vi "initialiseDevice.vi"(8 "error in (no error)":errorcluster, 10 "deviceName":string, 11 "AtomChipHWC in":refnum<class "AtomChipHWC.lvclass">) -> (0 "error out":errorcluster, 3 "AtomChipHWC out":refnum<class "AtomChipHWC.lvclass">)   [LabVIEW 2011, in "Hardware.lvlib" / "HWControllers.lvlib" / "AtomChipHWC.lvclass"]
doc: "Initialise a hardware device. \nI.e. set its initial channel states etc."
uses:
  AtomChipHWC.lvclass
  AtomChipHWC.lvclass/AtomChipHWC.ctl
  Channels/VoltOutput/AnalogOutput.lvclass
  Channels/Digital/DigitalOutput.lvclass
  Channels/DDSOutput/Generic/DDSOutput.lvclass
  Network Controllers/NetworkCamera/NetworkCamera.lvclass
  HWController.lvclass
  Tools/DatabaseHelpers/DbConnection/DeviceDataBase/deviceDataBase.lvclass
  Network Controllers/CameraNetworkController/CameraNetworkController.lvclass
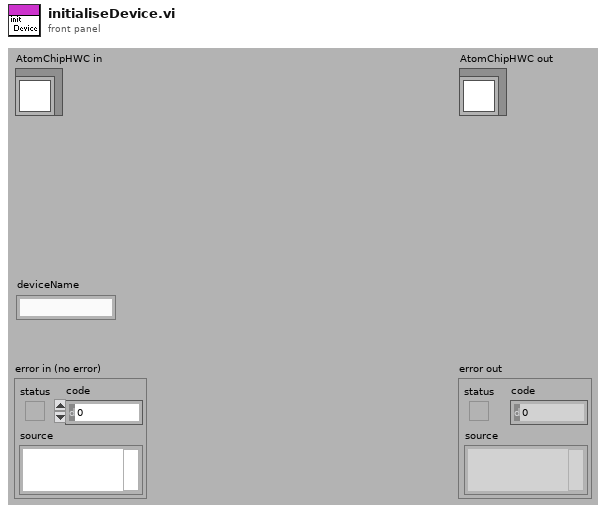
[diagram p1: front panel]
types:
  T1 = cluster{"VoltageLimit":dbl, "CurrentLimit":dbl}[]
  T2 = cluster{"Frequency(MHz)":dbl, "Amplitude":dbl, "Phase":dbl, "OutputForm":enum16{"Sine", "Square", "Triangle", "Arbitrary"}}[]
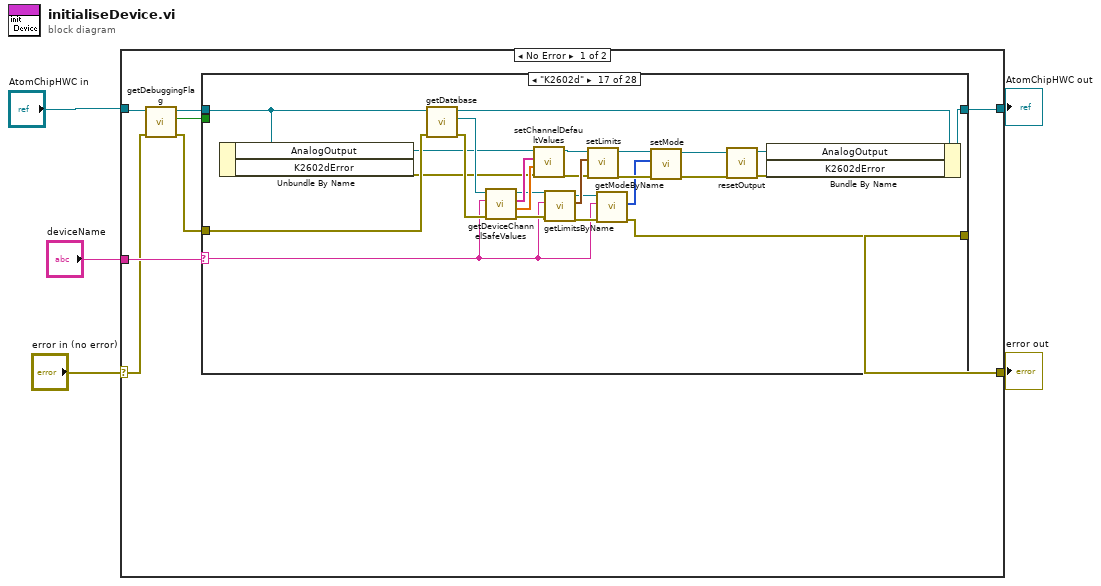
[diagram p0: block diagram]
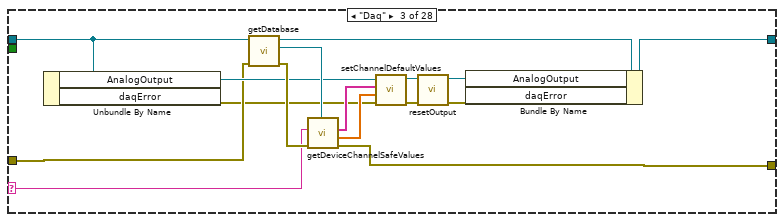
[diagram p4: hidden frame]
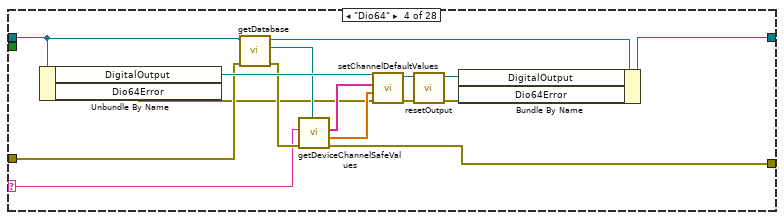
[diagram p5: hidden frame]
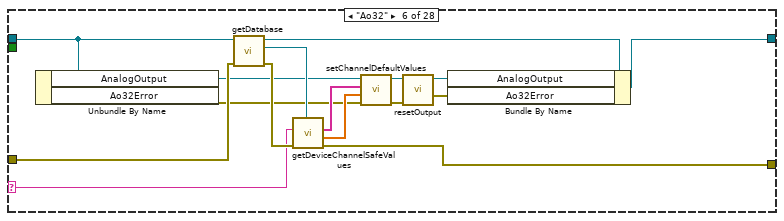
[diagram p7: hidden frame]
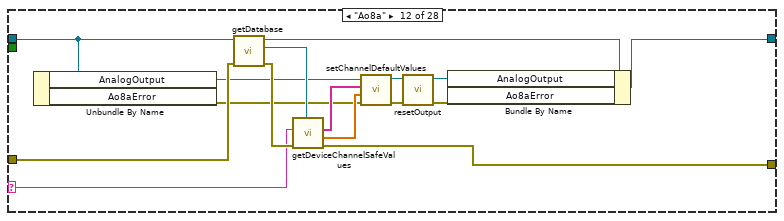
[diagram p13: hidden frame]
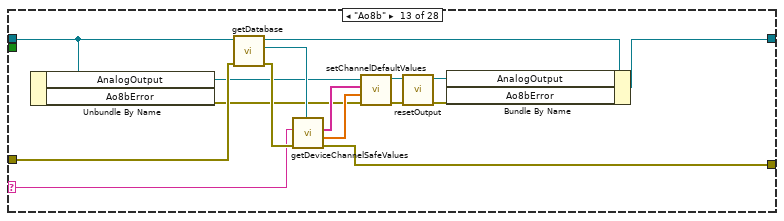
[diagram p14: hidden frame]
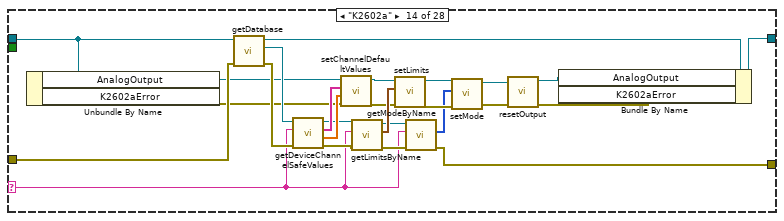
[diagram p15: hidden frame]
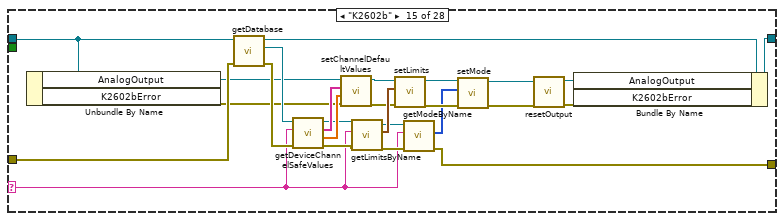
[diagram p16: hidden frame]
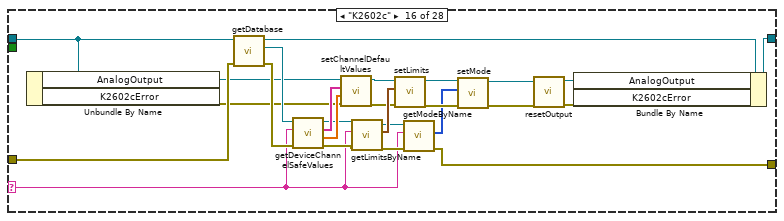
[diagram p17: hidden frame]
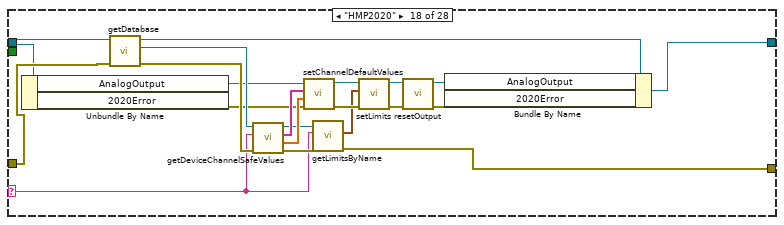
[diagram p18: hidden frame]
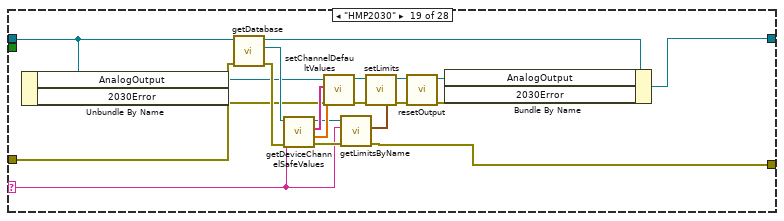
[diagram p19: hidden frame]
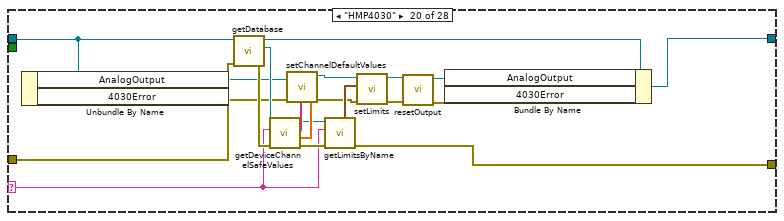
[diagram p20: hidden frame]
diagram:
  n1 = case shown="No Error" "error in (no error)" {
    selector: "error in (no error)" -> [w8 w374]
    tunnel: [w11 w374] -> w4
    tunnel: [w13 w373] -> w2
    tunnel: "AtomChipHWC in" -> [w10 w373]
    tunnel: "deviceName" -> [w12 _]
    frame No Error {
      n2 = call "getDebuggingFlag.vi"("error in (no error)"=w8, "HWController.lvclass in"=w10) -> ("error out"=w7:errorcluster, "debuggingFlag"=w6:bool, "HWController.lvclass out"=w9:refnum<class "AtomChipHWC.lvclass">)  [unwired: 7 in]
      n3 = case shown="\"K2602d\"" w12 {
        selector: w12 -> [_ _ w21 w40 _ w65 _ _ _ _ _ w91 w107 w112 w138 w164 w190 w220 w236 w257 w285 w302 w321 w339 _ _ _ _]
        tunnel: w9 -> [w15 w17 w24 w44 w50 w59 w69 w71 w73 w75 w77 w86 w101 w130 w156 w182 w208 w223 w251 w272 w291 w307 w325 w343 w350 w358 w365 w372]
        tunnel: [w15 w17 w22 w45 w50 w55 w69 w71 w73 w75 w77 w82 w97 w126 w152 w178 w204 w228 w247 w268 w289 w305 w323 w341 w348 w357 w364 w371] -> w13
        tunnel: w7 -> [w14 w16 w23 w37 w51 w64 w68 w70 w72 w74 w76 w90 w106 w133 w159 w185 w211 w232 w253 w274 w292 w308 w326 w344 w345 w356 w363 w370]
        tunnel: [w14 w16 w18 w34 w51 w52 w68 w70 w72 w74 w76 w79 w96 w110 w137 w163 w189 w219 w235 w256 w279 w295 w314 w332 w345 w356 w363 w370] -> w11
        tunnel: w6 -> [_ _ _ _ _ _ _ _ _ _ _ _ _ _ _ _ _ _ _ _ _ _ _ _ _ _ _ _]
        frame "No Hardware", Default {
        }
        frame "UsbDAQ" {
        }
        frame "Daq" {
          n4 = Unbundle By Name(w24) -> ("AnalogOutput"=w27:refnum<class "AnalogOutput.lvclass">, "daqError"=w20:errorcluster)
          n5 = call "getDatabase.vi"("error in (no error)"=w23, "HWController in"=w24) -> ("error out"=w32:errorcluster, "deviceDataBase"=w33:refnum<class "deviceDataBase.lvclass">, "HWController out"=w25:refnum<class "AtomChipHWC.lvclass">)  [unwired: 7 in]
          n6 = call "getDeviceChannelSafeValues.vi"("error in (no error)"=w32, "device_name"=w21, "deviceDataBase in"=w33) -> ("error out"=w18:errorcluster, "SafeVaues"=w31:dbl[], "ChannelAddresses"=w30:string[])  [unwired: 5 in, 1 out]
          n7 = call "setChannelDefaultValues.vi"("error in (no error)"=w20, "calibratedValues"=w31, "channel_addresses"=w30, "AnalogOutput in"=w27) -> ("error out"=w28:errorcluster, "AnalogOutput out"=w29:refnum<class "AnalogOutput.lvclass">)  [unwired: 6 in]
          n8 = call-dynamic "resetOutput.vi"("error in (no error)"=w28, "AnalogOutput in"=w29) -> ("error out"=w19:errorcluster, "AnalogOutput out"=w26:refnum<class "AnalogOutput.lvclass">)  [unwired: 8 in]
          n9 = Bundle By Name(cluster=w25, "AnalogOutput"=w26, "daqError"=w19) -> (w22:refnum<class "AtomChipHWC.lvclass">)
        }
        frame "Dio64" {
          n10 = Unbundle By Name(w44) -> ("DigitalOutput"=w49:refnum<class "DigitalOutput.lvclass">, "Dio64Error"=w36:errorcluster)
          n11 = call "getDatabase.vi"("error in (no error)"=w37, "HWController in"=w44) -> ("error out"=w41:errorcluster, "deviceDataBase"=w42:refnum<class "deviceDataBase.lvclass">, "HWController out"=w43:refnum<class "AtomChipHWC.lvclass">)  [unwired: 7 in]
          n12 = call "getDeviceChannelSafeValues.vi"("error in (no error)"=w41, "device_name"=w40, "deviceDataBase in"=w42) -> ("error out"=w34:errorcluster, "SafeVaues"=w38:dbl[], "ChannelAddresses"=w39:string[])  [unwired: 5 in, 1 out]
          n13 = call-dynamic "setChannelDefaultValues.vi"("error in (no error)"=w36, "calibratedValues"=w38, "channel_addresses"=w39, "DigitalOutput in"=w49) -> ("error out"=w47:errorcluster, "DigitalOutput out"=w48:refnum<class "DigitalOutput.lvclass">)  [unwired: 6 in]
          n14 = call-dynamic "resetOutput.vi"("error in (no error)"=w47, "DigitalOutput in"=w48) -> ("error out"=w35:errorcluster, "DigitalOutput out"=w46:refnum<class "DigitalOutput.lvclass">)  [unwired: 8 in]
          n15 = Bundle By Name(cluster=w43, "DigitalOutput"=w46, "Dio64Error"=w35) -> (w45:refnum<class "AtomChipHWC.lvclass">)
        }
        frame "Ao8" {
        }
        frame "Ao32" {
          n16 = Unbundle By Name(w59) -> ("AnalogOutput"=w58:refnum<class "AnalogOutput.lvclass">, "Ao32Error"=w54:errorcluster)
          n17 = call "getDatabase.vi"("error in (no error)"=w64, "HWController in"=w59) -> ("error out"=w66:errorcluster, "deviceDataBase"=w67:refnum<class "deviceDataBase.lvclass">, "HWController out"=w56:refnum<class "AtomChipHWC.lvclass">)  [unwired: 7 in]
          n18 = call "getDeviceChannelSafeValues.vi"("error in (no error)"=w66, "device_name"=w65, "deviceDataBase in"=w67) -> ("error out"=w52:errorcluster, "SafeVaues"=w63:dbl[], "ChannelAddresses"=w62:string[])  [unwired: 5 in, 1 out]
          n19 = call "setChannelDefaultValues.vi"("error in (no error)"=w54, "calibratedValues"=w63, "channel_addresses"=w62, "AnalogOutput in"=w58) -> ("error out"=w60:errorcluster, "AnalogOutput out"=w61:refnum<class "AnalogOutput.lvclass">)  [unwired: 6 in]
          n20 = call-dynamic "resetOutput.vi"("error in (no error)"=w60, "AnalogOutput in"=w61) -> ("error out"=w53:errorcluster, "AnalogOutput out"=w57:refnum<class "AnalogOutput.lvclass">)  [unwired: 8 in]
          n21 = Bundle By Name(cluster=w56, "AnalogOutput"=w57, "Ao32Error"=w53) -> (w55:refnum<class "AtomChipHWC.lvclass">)
        }
        frame "ArbWave" {
        }
        frame "ICCamera" {
        }
        frame "AndorIKon" {
        }
        frame "S1010" {
        }
        frame "C100" {
        }
        frame "Ao8a" {
          n22 = Unbundle By Name(w86) -> ("AnalogOutput"=w85:refnum<class "AnalogOutput.lvclass">, "Ao8aError"=w80:errorcluster)
          n23 = call "getDatabase.vi"("error in (no error)"=w90, "HWController in"=w86) -> ("error out"=w92:errorcluster, "deviceDataBase"=w93:refnum<class "deviceDataBase.lvclass">, "HWController out"=w83:refnum<class "AtomChipHWC.lvclass">)  [unwired: 7 in]
          n24 = call "getDeviceChannelSafeValues.vi"("error in (no error)"=w92, "device_name"=w91, "deviceDataBase in"=w93) -> ("error out"=w79:errorcluster, "SafeVaues"=w81:dbl[], "ChannelAddresses"=w89:string[])  [unwired: 5 in, 1 out]
          n25 = call "setChannelDefaultValues.vi"("error in (no error)"=w80, "calibratedValues"=w81, "channel_addresses"=w89, "AnalogOutput in"=w85) -> ("error out"=w87:errorcluster, "AnalogOutput out"=w88:refnum<class "AnalogOutput.lvclass">)  [unwired: 6 in]
          n26 = call-dynamic "resetOutput.vi"("error in (no error)"=w87, "AnalogOutput in"=w88) -> ("error out"=w78:errorcluster, "AnalogOutput out"=w84:refnum<class "AnalogOutput.lvclass">)  [unwired: 8 in]
          n27 = Bundle By Name(cluster=w83, "AnalogOutput"=w84, "Ao8aError"=w78) -> (w82:refnum<class "AtomChipHWC.lvclass">)
        }
        frame "Ao8b" {
          n28 = Unbundle By Name(w101) -> ("AnalogOutput"=w100:refnum<class "AnalogOutput.lvclass">, "Ao8bError"=w94:errorcluster)
          n29 = call "getDatabase.vi"("error in (no error)"=w106, "HWController in"=w101) -> ("error out"=w108:errorcluster, "deviceDataBase"=w109:refnum<class "deviceDataBase.lvclass">, "HWController out"=w98:refnum<class "AtomChipHWC.lvclass">)  [unwired: 7 in]
          n30 = call "getDeviceChannelSafeValues.vi"("error in (no error)"=w108, "device_name"=w107, "deviceDataBase in"=w109) -> ("error out"=w96:errorcluster, "SafeVaues"=w105:dbl[], "ChannelAddresses"=w104:string[])  [unwired: 5 in, 1 out]
          n31 = call "setChannelDefaultValues.vi"("error in (no error)"=w94, "calibratedValues"=w105, "channel_addresses"=w104, "AnalogOutput in"=w100) -> ("error out"=w102:errorcluster, "AnalogOutput out"=w103:refnum<class "AnalogOutput.lvclass">)  [unwired: 6 in]
          n32 = call-dynamic "resetOutput.vi"("error in (no error)"=w102, "AnalogOutput in"=w103) -> ("error out"=w95:errorcluster, "AnalogOutput out"=w99:refnum<class "AnalogOutput.lvclass">)  [unwired: 8 in]
          n33 = Bundle By Name(cluster=w98, "AnalogOutput"=w99, "Ao8bError"=w95) -> (w97:refnum<class "AtomChipHWC.lvclass">)
        }
        frame "K2602a" {
          n34 = Unbundle By Name(w130) -> ("AnalogOutput"=w129:refnum<class "AnalogOutput.lvclass">, "K2602aError"=w124:errorcluster)
          n35 = call "getDatabase.vi"("error in (no error)"=w133, "HWController in"=w130) -> ("error out"=w134:errorcluster, "deviceDataBase"=w135:refnum<class "deviceDataBase.lvclass">, "HWController out"=w127:refnum<class "AtomChipHWC.lvclass">)  [unwired: 7 in]
          n36 = call "getDeviceChannelSafeValues.vi"("error in (no error)"=w134, "device_name"=w112, "deviceDataBase in"=w135) -> ("error out"=w122:errorcluster, "SafeVaues"=w132:dbl[], "ChannelAddresses"=w131:string[], "deviceDataBase out"=w123:refnum<class "deviceDataBase.lvclass">)  [unwired: 5 in]
          n37 = call "setChannelDefaultValues.vi"("error in (no error)"=w124, "calibratedValues"=w132, "channel_addresses"=w131, "AnalogOutput in"=w129) -> ("error out"=w119:errorcluster, "AnalogOutput out"=w121:refnum<class "AnalogOutput.lvclass">)  [unwired: 6 in]
          n38 = call "getLimitsByName.vi"("error in (no error)"=w122, "device_name"=w112, "deviceDataBase in"=w123) -> ("error out"=w113:errorcluster, "Limits"=w120:T1, "deviceDataBase out"=w114:refnum<class "deviceDataBase.lvclass">)  [unwired: 6 in]
          n39 = call "setLimits.vi"("error in (no error)"=w119, "Limits"=w120, "AnalogOutput in"=w121) -> ("error out"=w115:errorcluster, "AnalogOutput out"=w118:refnum<class "AnalogOutput.lvclass">)  [unwired: 7 in]
          n40 = call "getModeByName.vi"("error in (no error)"=w113, "device_name"=w112, "deviceDataBase in"=w114) -> ("error out"=w110:errorcluster, "mode"=w111:enum16{"current", "voltage"}[])  [unwired: 6 in, 1 out]
          n41 = call "setMode.vi"("error in (no error)"=w115, "mode"=w111, "AnalogOutput in"=w118) -> ("error out"=w116:errorcluster, "AnalogOutput out"=w117:refnum<class "AnalogOutput.lvclass">)  [unwired: 7 in]
          n42 = call-dynamic "resetOutput.vi"("error in (no error)"=w116, "AnalogOutput in"=w117) -> ("error out"=w125:errorcluster, "AnalogOutput out"=w128:refnum<class "AnalogOutput.lvclass">)  [unwired: 8 in]
          n43 = Bundle By Name(cluster=w127, "AnalogOutput"=w128, "K2602aError"=w125) -> (w126:refnum<class "AtomChipHWC.lvclass">)
        }
        frame "K2602b" {
          n44 = Unbundle By Name(w156) -> ("AnalogOutput"=w155:refnum<class "AnalogOutput.lvclass">, "K2602bError"=w150:errorcluster)
          n45 = call "getDatabase.vi"("error in (no error)"=w159, "HWController in"=w156) -> ("error out"=w160:errorcluster, "deviceDataBase"=w161:refnum<class "deviceDataBase.lvclass">, "HWController out"=w153:refnum<class "AtomChipHWC.lvclass">)  [unwired: 7 in]
          n46 = call "getDeviceChannelSafeValues.vi"("error in (no error)"=w160, "device_name"=w138, "deviceDataBase in"=w161) -> ("error out"=w148:errorcluster, "SafeVaues"=w158:dbl[], "ChannelAddresses"=w157:string[], "deviceDataBase out"=w149:refnum<class "deviceDataBase.lvclass">)  [unwired: 5 in]
          n47 = call "setChannelDefaultValues.vi"("error in (no error)"=w150, "calibratedValues"=w158, "channel_addresses"=w157, "AnalogOutput in"=w155) -> ("error out"=w145:errorcluster, "AnalogOutput out"=w147:refnum<class "AnalogOutput.lvclass">)  [unwired: 6 in]
          n48 = call "getLimitsByName.vi"("error in (no error)"=w148, "device_name"=w138, "deviceDataBase in"=w149) -> ("error out"=w140:errorcluster, "Limits"=w146:T1, "deviceDataBase out"=w139:refnum<class "deviceDataBase.lvclass">)  [unwired: 6 in]
          n49 = call "setLimits.vi"("error in (no error)"=w145, "Limits"=w146, "AnalogOutput in"=w147) -> ("error out"=w143:errorcluster, "AnalogOutput out"=w144:refnum<class "AnalogOutput.lvclass">)  [unwired: 7 in]
          n50 = call "getModeByName.vi"("error in (no error)"=w140, "device_name"=w138, "deviceDataBase in"=w139) -> ("error out"=w137:errorcluster, "mode"=w136:enum16{"current", "voltage"}[])  [unwired: 6 in, 1 out]
          n51 = call "setMode.vi"("error in (no error)"=w143, "mode"=w136, "AnalogOutput in"=w144) -> ("error out"=w142:errorcluster, "AnalogOutput out"=w141:refnum<class "AnalogOutput.lvclass">)  [unwired: 7 in]
          n52 = call-dynamic "resetOutput.vi"("error in (no error)"=w142, "AnalogOutput in"=w141) -> ("error out"=w151:errorcluster, "AnalogOutput out"=w154:refnum<class "AnalogOutput.lvclass">)  [unwired: 8 in]
          n53 = Bundle By Name(cluster=w153, "AnalogOutput"=w154, "K2602bError"=w151) -> (w152:refnum<class "AtomChipHWC.lvclass">)
        }
        frame "K2602c" {
          n54 = Unbundle By Name(w182) -> ("AnalogOutput"=w181:refnum<class "AnalogOutput.lvclass">, "K2602cError"=w176:errorcluster)
          n55 = call "getDatabase.vi"("error in (no error)"=w185, "HWController in"=w182) -> ("error out"=w186:errorcluster, "deviceDataBase"=w187:refnum<class "deviceDataBase.lvclass">, "HWController out"=w179:refnum<class "AtomChipHWC.lvclass">)  [unwired: 7 in]
          n56 = call "getDeviceChannelSafeValues.vi"("error in (no error)"=w186, "device_name"=w164, "deviceDataBase in"=w187) -> ("error out"=w174:errorcluster, "SafeVaues"=w184:dbl[], "ChannelAddresses"=w183:string[], "deviceDataBase out"=w175:refnum<class "deviceDataBase.lvclass">)  [unwired: 5 in]
          n57 = call "setChannelDefaultValues.vi"("error in (no error)"=w176, "calibratedValues"=w184, "channel_addresses"=w183, "AnalogOutput in"=w181) -> ("error out"=w171:errorcluster, "AnalogOutput out"=w173:refnum<class "AnalogOutput.lvclass">)  [unwired: 6 in]
          n58 = call "getLimitsByName.vi"("error in (no error)"=w174, "device_name"=w164, "deviceDataBase in"=w175) -> ("error out"=w166:errorcluster, "Limits"=w172:T1, "deviceDataBase out"=w165:refnum<class "deviceDataBase.lvclass">)  [unwired: 6 in]
          n59 = call "setLimits.vi"("error in (no error)"=w171, "Limits"=w172, "AnalogOutput in"=w173) -> ("error out"=w169:errorcluster, "AnalogOutput out"=w170:refnum<class "AnalogOutput.lvclass">)  [unwired: 7 in]
          n60 = call "getModeByName.vi"("error in (no error)"=w166, "device_name"=w164, "deviceDataBase in"=w165) -> ("error out"=w163:errorcluster, "mode"=w162:enum16{"current", "voltage"}[])  [unwired: 6 in, 1 out]
          n61 = call "setMode.vi"("error in (no error)"=w169, "mode"=w162, "AnalogOutput in"=w170) -> ("error out"=w168:errorcluster, "AnalogOutput out"=w167:refnum<class "AnalogOutput.lvclass">)  [unwired: 7 in]
          n62 = call-dynamic "resetOutput.vi"("error in (no error)"=w168, "AnalogOutput in"=w167) -> ("error out"=w177:errorcluster, "AnalogOutput out"=w180:refnum<class "AnalogOutput.lvclass">)  [unwired: 8 in]
          n63 = Bundle By Name(cluster=w179, "AnalogOutput"=w180, "K2602cError"=w177) -> (w178:refnum<class "AtomChipHWC.lvclass">)
        }
        frame "K2602d" {
          n64 = Unbundle By Name(w208) -> ("AnalogOutput"=w207:refnum<class "AnalogOutput.lvclass">, "K2602dError"=w202:errorcluster)
          n65 = call "getDatabase.vi"("error in (no error)"=w211, "HWController in"=w208) -> ("error out"=w212:errorcluster, "deviceDataBase"=w213:refnum<class "deviceDataBase.lvclass">, "HWController out"=w205:refnum<class "AtomChipHWC.lvclass">)  [unwired: 7 in]
          n66 = call "getDeviceChannelSafeValues.vi"("error in (no error)"=w212, "device_name"=w190, "deviceDataBase in"=w213) -> ("error out"=w200:errorcluster, "SafeVaues"=w210:dbl[], "ChannelAddresses"=w209:string[], "deviceDataBase out"=w201:refnum<class "deviceDataBase.lvclass">)  [unwired: 5 in]
          n67 = call "setChannelDefaultValues.vi"("error in (no error)"=w202, "calibratedValues"=w210, "channel_addresses"=w209, "AnalogOutput in"=w207) -> ("error out"=w197:errorcluster, "AnalogOutput out"=w199:refnum<class "AnalogOutput.lvclass">)  [unwired: 6 in]
          n68 = call "getLimitsByName.vi"("error in (no error)"=w200, "device_name"=w190, "deviceDataBase in"=w201) -> ("error out"=w192:errorcluster, "Limits"=w198:T1, "deviceDataBase out"=w191:refnum<class "deviceDataBase.lvclass">)  [unwired: 6 in]
          n69 = call "setLimits.vi"("error in (no error)"=w197, "Limits"=w198, "AnalogOutput in"=w199) -> ("error out"=w195:errorcluster, "AnalogOutput out"=w196:refnum<class "AnalogOutput.lvclass">)  [unwired: 7 in]
          n70 = call "getModeByName.vi"("error in (no error)"=w192, "device_name"=w190, "deviceDataBase in"=w191) -> ("error out"=w189:errorcluster, "mode"=w188:enum16{"current", "voltage"}[])  [unwired: 6 in, 1 out]
          n71 = call "setMode.vi"("error in (no error)"=w195, "mode"=w188, "AnalogOutput in"=w196) -> ("error out"=w194:errorcluster, "AnalogOutput out"=w193:refnum<class "AnalogOutput.lvclass">)  [unwired: 7 in]
          n72 = call-dynamic "resetOutput.vi"("error in (no error)"=w194, "AnalogOutput in"=w193) -> ("error out"=w203:errorcluster, "AnalogOutput out"=w206:refnum<class "AnalogOutput.lvclass">)  [unwired: 8 in]
          n73 = Bundle By Name(cluster=w205, "AnalogOutput"=w206, "K2602dError"=w203) -> (w204:refnum<class "AtomChipHWC.lvclass">)
        }
        frame "HMP2020" {
          n74 = Unbundle By Name(w223) -> ("AnalogOutput"=w230:refnum<class "AnalogOutput.lvclass">, "2020Error"=w226:errorcluster)
          n75 = call "getDatabase.vi"("error in (no error)"=w232, "HWController in"=w223) -> ("error out"=w233:errorcluster, "deviceDataBase"=w234:refnum<class "deviceDataBase.lvclass">, "HWController out"=w224:refnum<class "AtomChipHWC.lvclass">)  [unwired: 7 in]
          n76 = call "getDeviceChannelSafeValues.vi"("error in (no error)"=w233, "device_name"=w220, "deviceDataBase in"=w234) -> ("error out"=w221:errorcluster, "SafeVaues"=w227:dbl[], "ChannelAddresses"=w231:string[], "deviceDataBase out"=w222:refnum<class "deviceDataBase.lvclass">)  [unwired: 5 in]
          n77 = call "setChannelDefaultValues.vi"("error in (no error)"=w226, "calibratedValues"=w227, "channel_addresses"=w231, "AnalogOutput in"=w230) -> ("error out"=w216:errorcluster, "AnalogOutput out"=w218:refnum<class "AnalogOutput.lvclass">)  [unwired: 6 in]
          n78 = call "getLimitsByName.vi"("error in (no error)"=w221, "device_name"=w220, "deviceDataBase in"=w222) -> ("error out"=w219:errorcluster, "Limits"=w214:T1)  [unwired: 6 in, 1 out]
          n79 = call "setLimits.vi"("error in (no error)"=w216, "Limits"=w214, "AnalogOutput in"=w218) -> ("error out"=w215:errorcluster, "AnalogOutput out"=w217:refnum<class "AnalogOutput.lvclass">)  [unwired: 7 in]
          n80 = call-dynamic "resetOutput.vi"("error in (no error)"=w215, "AnalogOutput in"=w217) -> ("error out"=w225:errorcluster, "AnalogOutput out"=w229:refnum<class "AnalogOutput.lvclass">)  [unwired: 8 in]
          n81 = Bundle By Name(cluster=w224, "AnalogOutput"=w229, "2020Error"=w225) -> (w228:refnum<class "AtomChipHWC.lvclass">)
        }
        frame "HMP2030" {
          n82 = Unbundle By Name(w251) -> ("AnalogOutput"=w250:refnum<class "AnalogOutput.lvclass">, "2030Error"=w245:errorcluster)
          n83 = call "getDatabase.vi"("error in (no error)"=w253, "HWController in"=w251) -> ("error out"=w254:errorcluster, "deviceDataBase"=w255:refnum<class "deviceDataBase.lvclass">, "HWController out"=w248:refnum<class "AtomChipHWC.lvclass">)  [unwired: 7 in]
          n84 = call "getDeviceChannelSafeValues.vi"("error in (no error)"=w254, "device_name"=w236, "deviceDataBase in"=w255) -> ("error out"=w237:errorcluster, "SafeVaues"=w246:dbl[], "ChannelAddresses"=w252:string[], "deviceDataBase out"=w238:refnum<class "deviceDataBase.lvclass">)  [unwired: 5 in]
          n85 = call "setChannelDefaultValues.vi"("error in (no error)"=w245, "calibratedValues"=w246, "channel_addresses"=w252, "AnalogOutput in"=w250) -> ("error out"=w239:errorcluster, "AnalogOutput out"=w242:refnum<class "AnalogOutput.lvclass">)  [unwired: 6 in]
          n86 = call "getLimitsByName.vi"("error in (no error)"=w237, "device_name"=w236, "deviceDataBase in"=w238) -> ("error out"=w235:errorcluster, "Limits"=w243:T1)  [unwired: 6 in, 1 out]
          n87 = call "setLimits.vi"("error in (no error)"=w239, "Limits"=w243, "AnalogOutput in"=w242) -> ("error out"=w240:errorcluster, "AnalogOutput out"=w241:refnum<class "AnalogOutput.lvclass">)  [unwired: 7 in]
          n88 = call-dynamic "resetOutput.vi"("error in (no error)"=w240, "AnalogOutput in"=w241) -> ("error out"=w244:errorcluster, "AnalogOutput out"=w249:refnum<class "AnalogOutput.lvclass">)  [unwired: 8 in]
          n89 = Bundle By Name(cluster=w248, "AnalogOutput"=w249, "2030Error"=w244) -> (w247:refnum<class "AtomChipHWC.lvclass">)
        }
        frame "HMP4030" {
          n90 = Unbundle By Name(w272) -> ("AnalogOutput"=w271:refnum<class "AnalogOutput.lvclass">, "4030Error"=w266:errorcluster)
          n91 = call "getDatabase.vi"("error in (no error)"=w274, "HWController in"=w272) -> ("error out"=w275:errorcluster, "deviceDataBase"=w276:refnum<class "deviceDataBase.lvclass">, "HWController out"=w269:refnum<class "AtomChipHWC.lvclass">)  [unwired: 7 in]
          n92 = call "getDeviceChannelSafeValues.vi"("error in (no error)"=w275, "device_name"=w257, "deviceDataBase in"=w276) -> ("error out"=w259:errorcluster, "SafeVaues"=w267:dbl[], "ChannelAddresses"=w273:string[], "deviceDataBase out"=w258:refnum<class "deviceDataBase.lvclass">)  [unwired: 5 in]
          n93 = call "setChannelDefaultValues.vi"("error in (no error)"=w266, "calibratedValues"=w267, "channel_addresses"=w273, "AnalogOutput in"=w271) -> ("error out"=w260:errorcluster, "AnalogOutput out"=w263:refnum<class "AnalogOutput.lvclass">)  [unwired: 6 in]
          n94 = call "getLimitsByName.vi"("error in (no error)"=w259, "device_name"=w257, "deviceDataBase in"=w258) -> ("error out"=w256:errorcluster, "Limits"=w264:T1)  [unwired: 6 in, 1 out]
          n95 = call "setLimits.vi"("error in (no error)"=w260, "Limits"=w264, "AnalogOutput in"=w263) -> ("error out"=w261:errorcluster, "AnalogOutput out"=w262:refnum<class "AnalogOutput.lvclass">)  [unwired: 7 in]
          n96 = call-dynamic "resetOutput.vi"("error in (no error)"=w261, "AnalogOutput in"=w262) -> ("error out"=w265:errorcluster, "AnalogOutput out"=w270:refnum<class "AnalogOutput.lvclass">)  [unwired: 8 in]
          n97 = Bundle By Name(cluster=w269, "AnalogOutput"=w270, "4030Error"=w265) -> (w268:refnum<class "AtomChipHWC.lvclass">)
        }
        frame "SpinCoreDDS0" {
          n98 = Unbundle By Name(w291) -> ("DDSOutput"=w288:refnum<class "DDSOutput.lvclass">, "DDS0Error"=w278:errorcluster)
          n99 = call "getDatabase.vi"("error in (no error)"=w292, "HWController in"=w291) -> ("error out"=w287:errorcluster, "deviceDataBase"=w286:refnum<class "deviceDataBase.lvclass">, "HWController out"=w290:refnum<class "AtomChipHWC.lvclass">)  [unwired: 7 in]
          n100 = call "getRfChannelSafeStates.vi"("error in (no error)"=w287, "deviceName"=w285, "deviceDataBase in"=w286) -> ("error out"=w279:errorcluster, "safestates"=w280:T2, "ChannelAddresses"=w281:string[])  [unwired: 5 in, 1 out]
          n101 = call-dynamic "setChannelDefaults.vi"("error in (no error)"=w278, "Data"=w280, "physicalChannels"=w281, "DDSOutput in"=w288) -> ("error out"=w282:errorcluster, "DDSOutput out"=w284:refnum<class "DDSOutput.lvclass">)  [unwired: 6 in]
          n102 = call-dynamic "resetOutput.vi"("error in (no error)"=w282, "DDSOutput in"=w284) -> ("error out"=w277:errorcluster, "DDSOutput out"=w283:refnum<class "DDSOutput.lvclass">)  [unwired: 8 in]
          n103 = Bundle By Name(cluster=w290, "DDSOutput"=w283, "DDS0Error"=w277) -> (w289:refnum<class "AtomChipHWC.lvclass">)
        }
        frame "SpinCoreDDS1" {
          n104 = Unbundle By Name(w307) -> ("DDSOutput"=w304:refnum<class "DDSOutput.lvclass">, "DDS1Error"=w294:errorcluster)
          n105 = call "getDatabase.vi"("error in (no error)"=w308, "HWController in"=w307) -> ("error out"=w303:errorcluster, "deviceDataBase"=w301:refnum<class "deviceDataBase.lvclass">, "HWController out"=w306:refnum<class "AtomChipHWC.lvclass">)  [unwired: 7 in]
          n106 = call "getRfChannelSafeStates.vi"("error in (no error)"=w303, "deviceName"=w302, "deviceDataBase in"=w301) -> ("error out"=w295:errorcluster, "safestates"=w299:T2, "ChannelAddresses"=w300:string[])  [unwired: 5 in, 1 out]
          n107 = call-dynamic "setChannelDefaults.vi"("error in (no error)"=w294, "Data"=w299, "physicalChannels"=w300, "DDSOutput in"=w304) -> ("error out"=w296:errorcluster, "DDSOutput out"=w298:refnum<class "DDSOutput.lvclass">)  [unwired: 6 in]
          n108 = call-dynamic "resetOutput.vi"("error in (no error)"=w296, "DDSOutput in"=w298) -> ("error out"=w293:errorcluster, "DDSOutput out"=w297:refnum<class "DDSOutput.lvclass">)  [unwired: 8 in]
          n109 = Bundle By Name(cluster=w306, "DDSOutput"=w297, "DDS1Error"=w293) -> (w305:refnum<class "AtomChipHWC.lvclass">)
        }
        frame "k3390" {
          n110 = Unbundle By Name(w325) -> ("DDSOutput"=w311:refnum<class "DDSOutput.lvclass">, "DDS1Error"=w309:errorcluster)
          n111 = call "getDatabase.vi"("error in (no error)"=w326, "HWController in"=w325) -> ("error out"=w322:errorcluster, "deviceDataBase"=w320:refnum<class "deviceDataBase.lvclass">, "HWController out"=w324:refnum<class "AtomChipHWC.lvclass">)  [unwired: 7 in]
          n112 = call "getRfChannelSafeStates.vi"("error in (no error)"=w322, "deviceName"=w321, "deviceDataBase in"=w320) -> ("error out"=w314:errorcluster, "safestates"=w318:T2, "ChannelAddresses"=w319:string[])  [unwired: 5 in, 1 out]
          n113 = call-dynamic "initialise.vi"("error in (no error)"=w309, "DDSOutput in"=w311) -> ("error out"=w310:errorcluster, "DDSOutput out"=w312:refnum<class "DDSOutput.lvclass">)  [unwired: 8 in]
          n114 = call-dynamic "setChannelDefaults.vi"("error in (no error)"=w310, "Data"=w318, "physicalChannels"=w319, "DDSOutput in"=w312) -> ("error out"=w315:errorcluster, "DDSOutput out"=w317:refnum<class "DDSOutput.lvclass">)  [unwired: 6 in]
          n115 = call-dynamic "resetOutput.vi"("error in (no error)"=w315, "DDSOutput in"=w317) -> ("error out"=w313:errorcluster, "DDSOutput out"=w316:refnum<class "DDSOutput.lvclass">)  [unwired: 8 in]
          n116 = Bundle By Name(cluster=w324, "DDSOutput"=w316, "DDS1Error"=w313) -> (w323:refnum<class "AtomChipHWC.lvclass">)
        }
        frame "CQTDDS0" {
          n117 = Unbundle By Name(w343) -> ("DDSOutput"=w329:refnum<class "DDSOutput.lvclass">, "DDS0Error"=w327:errorcluster)
          n118 = call "getDatabase.vi"("error in (no error)"=w344, "HWController in"=w343) -> ("error out"=w340:errorcluster, "deviceDataBase"=w338:refnum<class "deviceDataBase.lvclass">, "HWController out"=w342:refnum<class "AtomChipHWC.lvclass">)  [unwired: 7 in]
          n119 = call "getRfChannelSafeStates.vi"("error in (no error)"=w340, "deviceName"=w339, "deviceDataBase in"=w338) -> ("error out"=w332:errorcluster, "safestates"=w336:T2, "ChannelAddresses"=w337:string[])  [unwired: 5 in, 1 out]
          n120 = call-dynamic "initialise.vi"("error in (no error)"=w327, "DDSOutput in"=w329) -> ("error out"=w328:errorcluster, "DDSOutput out"=w330:refnum<class "DDSOutput.lvclass">)  [unwired: 8 in]
          n121 = call-dynamic "setChannelDefaults.vi"("error in (no error)"=w328, "Data"=w336, "physicalChannels"=w337, "DDSOutput in"=w330) -> ("error out"=w333:errorcluster, "DDSOutput out"=w335:refnum<class "DDSOutput.lvclass">)  [unwired: 6 in]
          n122 = call-dynamic "resetOutput.vi"("error in (no error)"=w333, "DDSOutput in"=w335) -> ("error out"=w331:errorcluster, "DDSOutput out"=w334:refnum<class "DDSOutput.lvclass">)  [unwired: 8 in]
          n123 = Bundle By Name(cluster=w342, "DDSOutput"=w334, "DDS0Error"=w331) -> (w341:refnum<class "AtomChipHWC.lvclass">)
        }
        frame "oldPixelfly", "oldProEM_WinX32" {
          n124 = Unbundle By Name(w350) -> ("CameraNetworkController"=w351:refnum<class "CameraNetworkController.lvclass">, "CameraNError"=w347:errorcluster)
          n125 = call "initialise.vi"("error in (no error)"=w347, "CameraNetworkController in"=w351) -> ("error out"=w346:errorcluster, "CameraNetworkController out"=w349:refnum<class "CameraNetworkController.lvclass">)  [unwired: 8 in]
          n126 = Bundle By Name(cluster=w350, "CameraNetworkController"=w349, "CameraNError"=w346) -> (w348:refnum<class "AtomChipHWC.lvclass">)
        }
        frame "Pixelfly" {
          n127 = Unbundle By Name(w358) -> ("netCam"=w355:refnum<class "NetworkCamera.lvclass">, "netCamError"=w353:errorcluster)
          n128 = call-dynamic "initialise.vi"("error in (no error)"=w353, "NetworkCamera in"=w355) -> ("error out"=w352:errorcluster, "NetworkCamera out"=w354:refnum<class "NetworkCamera.lvclass">)  [unwired: 8 in]
          n129 = Bundle By Name(cluster=w358, "netCam"=w354, "netCamError"=w352) -> (w357:refnum<class "AtomChipHWC.lvclass">)
        }
        frame "Pixis" {
          n130 = Unbundle By Name(w365) -> ("netCam"=w362:refnum<class "NetworkCamera.lvclass">, "netCamError"=w360:errorcluster)
          n131 = call-dynamic "initialise.vi"("error in (no error)"=w360, "NetworkCamera in"=w362) -> ("error out"=w359:errorcluster, "NetworkCamera out"=w361:refnum<class "NetworkCamera.lvclass">)  [unwired: 8 in]
          n132 = Bundle By Name(cluster=w365, "netCam"=w361, "netCamError"=w359) -> (w364:refnum<class "AtomChipHWC.lvclass">)
        }
        frame "ProEM" {
          n133 = Unbundle By Name(w372) -> ("netCam"=w369:refnum<class "NetworkCamera.lvclass">, "netCamError"=w367:errorcluster)
          n134 = call-dynamic "initialise.vi"("error in (no error)"=w367, "NetworkCamera in"=w369) -> ("error out"=w366:errorcluster, "NetworkCamera out"=w368:refnum<class "NetworkCamera.lvclass">)  [unwired: 8 in]
          n135 = Bundle By Name(cluster=w372, "netCam"=w368, "netCamError"=w366) -> (w371:refnum<class "AtomChipHWC.lvclass">)
        }
      }
    }
    frame Error {
    }
  }
  "error out" <- w4
  "AtomChipHWC out" <- w2
